vi "best_angle.vi"(3 "Waypoint Heading":dbl, 4 "Current Heading":dbl) -> (0 "Heading Candidate 2":dbl, 1 "Heading Candidate 1":dbl, 2 "Best Angle":dbl)   [LabVIEW 2011]
doc: "Takes the absolute wind vector, the heading of your next waypoint, and your current heading, and recommends a heading.\n\nWe repeatedly run the iterate theta VI until its outputs converge. The converging outputs are the two angles which minimize the travel time to the waypoint.\n\nAfter the while loop, we determine which angle is closer to the current heading. We choose the closer heading unless the other heading has a significantly higher dr/dt."
uses:
  2 Globals/2 Global.vi
panel:
  in  "thres+":dbl=2.0
  in  "thresh x":dbl=1.2
  # "Inputs"
  # "Outputs"
  # "Constants to determine when to tack"
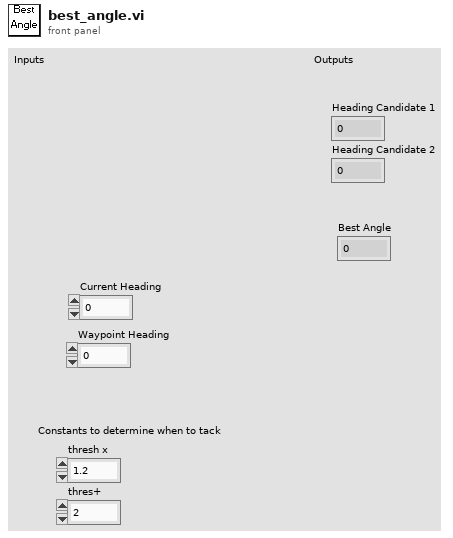
[diagram p1: front panel]
types:
  T1 = typedef "apparent wind direction.ctl" = dbl
  T2 = typedef "apparent wind speed.ctl" = dbl
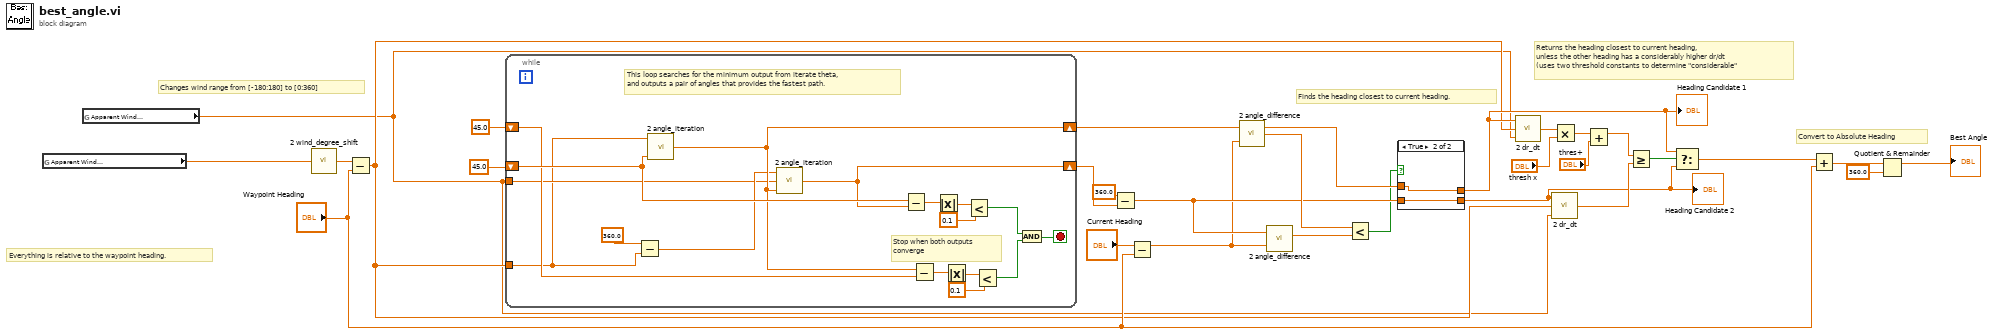
[diagram p0: block diagram]
diagram:
  # "Returns the heading closest to current heading,\nunless the other heading has a considerably higher dr/dt\n(uses two threshold constants to determine \"considerable\""
  # "Finds the heading closest to current heading."
  # "Changes wind range from [-180:180] to [0:360]"
  # "Convert to Absolute Heading"
  # "Everything is relative to the waypoint heading."
  n1 = global read "2 Global.vi" "Apparent Wind\nDirection (º)"() -> (w1:T1)
  n2 = global read "2 Global.vi" "Apparent Wind\nSpeed"() -> (w2:T2)
  n3 = call "2 wind_degree_shift.vi"("Wind Theta -180 - 180"=w1) -> ("Wind Theta 0-360"=w4:dbl)
  n4 = Subtract(x=w4, y="Waypoint Heading") -> (x-y=w3:dbl)
  n5 = while {
    shift-right: [w42] -> w25
    shift-left: 45.0 ("Best Theta") -> [w43]
    shift-right: [w33] -> w16
    shift-left: 45.0 ("Best Theta") -> [w38]
    tunnel: w3 -> [w30]
    tunnel: w2 -> [w31]
    stop <- w35 stop-if-true
    # "This loop searches for the minimum output from iterate theta,\nand outputs a pair of angles that provides the fastest path."
    # "Stop when both outputs\nconverge"
    n6 = Subtract(x=360.0, y=w30) -> (x-y=w32:dbl)
    n7 = call "2 angle_iteration.vi"("Phi"=w43, "Apparent Wind\nDirection (º)"=w30) -> ("Best Theta"=w33:dbl)  [unwired: 1 in]
    n8 = call "2 angle_iteration.vi"("Phi"=w33, "Apparent Wind\nSpeed"=w31, "Apparent Wind\nDirection (º)"=w32) -> ("Best Theta"=w42:dbl)
    n9 = Subtract(x=w43, y=w42) -> (x-y=w46:dbl)
    n10 = Subtract(x=w33, y=w38) -> (x-y=w39:dbl)
    n11 = Absolute Value(x=w46) -> (abs(x)=w45:dbl)
    n12 = Absolute Value(x=w39) -> (abs(x)=w40:dbl)
    n13 = Less?(x=w45, y=0.1) -> (x < y?=w37:bool)
    n14 = Less?(x=w40, y=0.1) -> (x < y?=w36:bool)
    n15 = And(x=w37, y=w36) -> (x .and. y?=w35:bool)
  }
  n16 = Subtract(x=360.0, y=w25) -> (x-y=w15:dbl)
  n17 = Subtract(x="Current Heading", y="Waypoint Heading") -> (x-y=w11:dbl)
  n18 = call "2 angle_difference.vi"("Angle 2"=w11, "Angle 1"=w16) -> ("Difference"=w23:dbl)
  n19 = call "2 angle_difference.vi"("Angle 2"=w11, "Angle 1"=w15) -> ("Difference"=w24:dbl)
  n20 = Less?(x=w23, y=w24) -> (x < y?=w14:bool)
  n21 = case shown="True" w14 {
    tunnel: w16 -> [w48 w50]
    tunnel: [w47 w50] -> w6
    tunnel: [w48 w49] -> w5
    tunnel: w15 -> [w47 w49]
    frame False {
    }
    frame True {
    }
  }
  "Heading Candidate 1" <- w6
  "Heading Candidate 2" <- w5
  n22 = call "2 dr_dt.vi"("Apparent Wind\nSpeed"=w2, "Apparent Wind\nDirection (º)"=w3, "Boat Angle"=w6) -> ("dr/dt"=w21:dbl)
  n23 = call "2 dr_dt.vi"("Apparent Wind\nSpeed"=w2, "Apparent Wind\nDirection (º)"=w3, "Boat Angle"=w5) -> ("dr/dt"=w18:dbl)
  n24 = Multiply(x=w21, y="thresh x") -> (x*y=w17:dbl)
  n25 = Add(x=w17, y="thres+") -> (x+y=w13:dbl)
  n26 = Greater Or Equal?(x=w13, y=w18) -> (x >= y?=w19:bool)
  n27 = Select(t=w6, s=w19, f=w5) -> (s? t:f=w28:dbl)
  n28 = Add(x=w28, y="Waypoint Heading") -> (x+y=w9:dbl)
  n29 = Quotient & Remainder(x=w9, y=360.0) -> (x-y*floor(x/y)=→"Best Angle":dbl)  [unwired: 1 out]
